vi "PWM_Mearsurement.vi"() -> ()   [LabVIEW 2019]
uses:
  <vilib>/rvi/Emulation/niFpgaGetClockAttributes.vi
  <vilib>/rvi/Emulation/niFpgaSctlEmulationGetInTimedLoop.vi
  <vilib>/rvi/Emulation/niFpgaEmulationReportErrorSimple.vi
  <vilib>/rvi/eio/common/nirviEmuTemplateMethod_errors.vi
  <vilib>/rvi/Emulation/niFpgaCriticalErrorInLSC.vi
  <vilib>/eio/EIONode/EIONode.xnode
panel:
  out "波形图表 3":cluster{u32, u32}(graph)
  out "时钟信号个数 3":u32
  out "被测信号个数 3":u32
  in  "Count(Ticks) 3":u32=16 caption="计数器(滴答)"
  out "波形图表 2":cluster{u32, u32}(graph)
  out "被测信号个数 2":u32
  out "时钟信号个数 2":u32
  in  "Count(Ticks) 2":u32=16 caption="计数器(滴答)"
  out "被测信号个数":u32
  out "时钟信号个数":u32
  out "x+1":u32
  out "数值":u32
  in  "Count(Ticks)":u32=16 caption="计数器(滴答)"
  out "x-1":u32
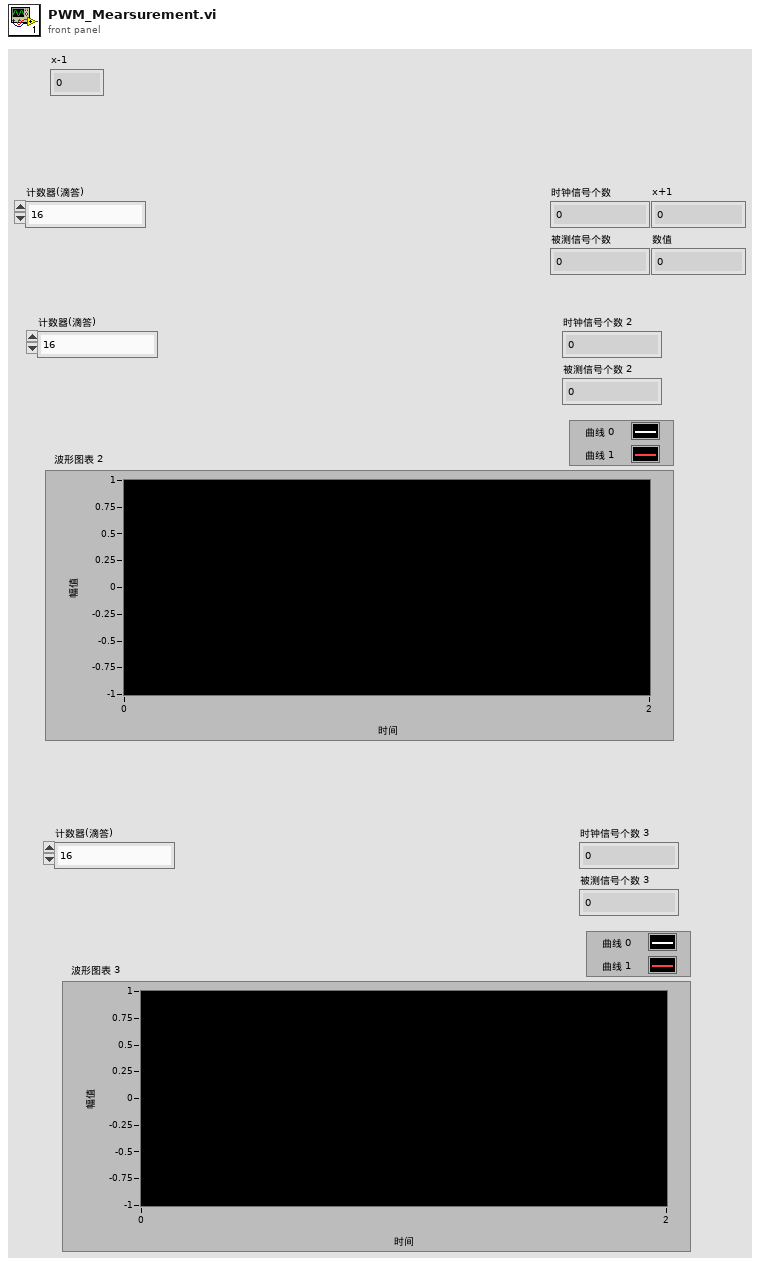
[diagram p1: front panel]
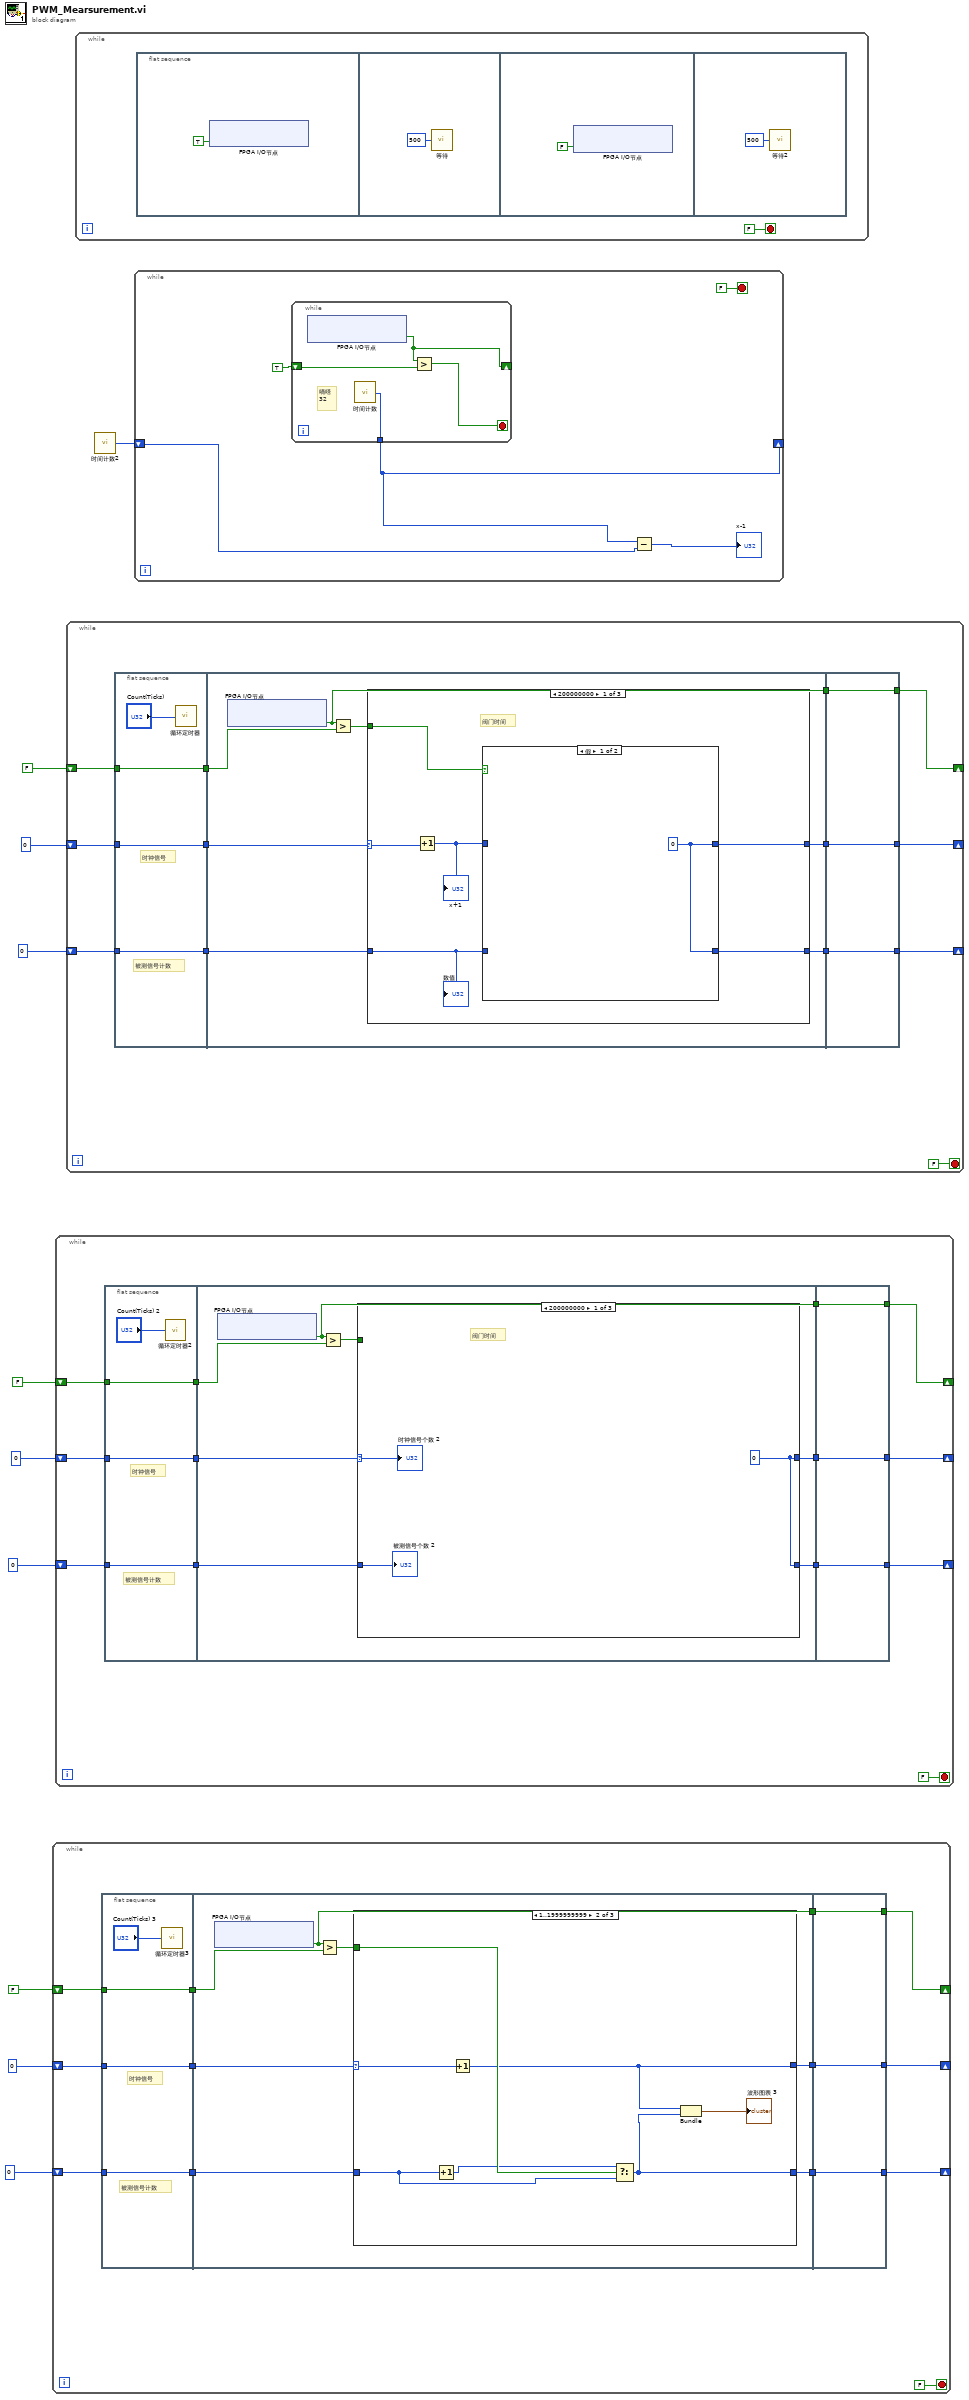
[diagram p0: block diagram]
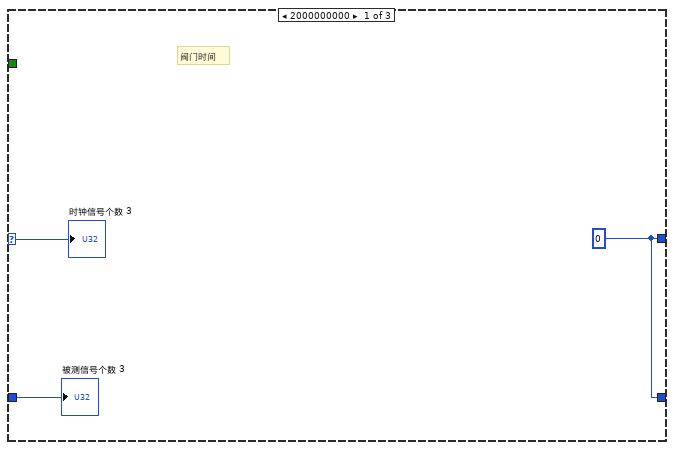
[diagram p2: hidden frame]
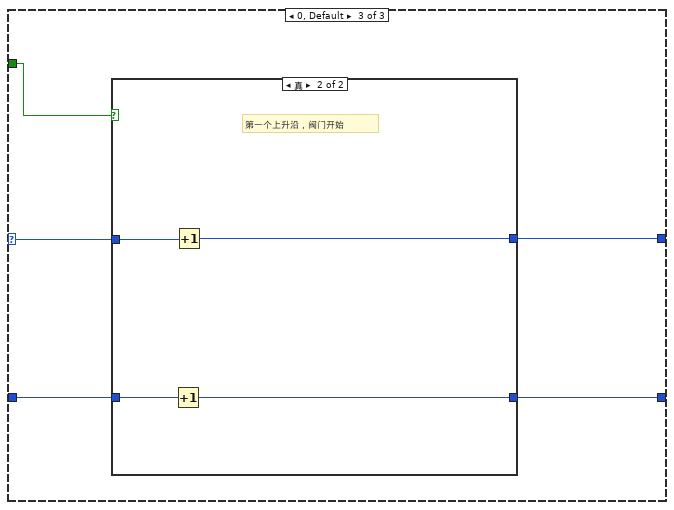
[diagram p3: hidden frame]
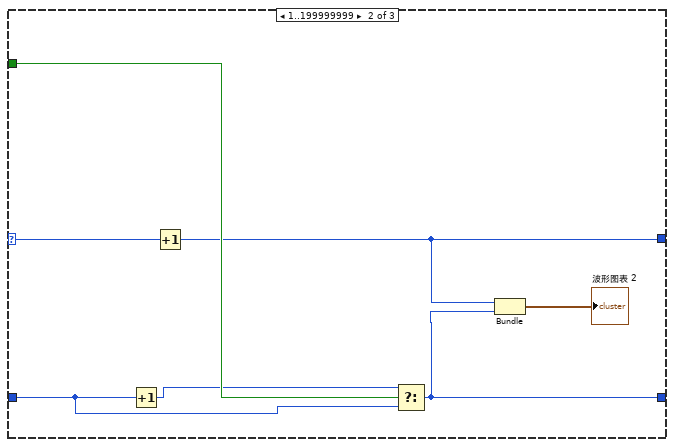
[diagram p5: hidden frame]
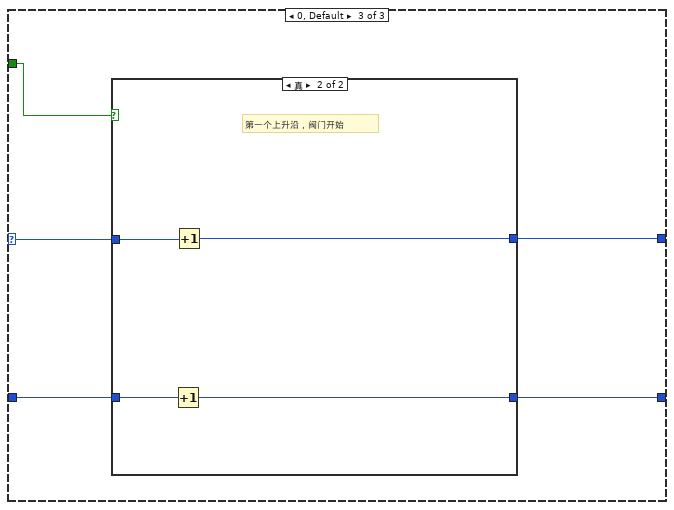
[diagram p6: hidden frame]
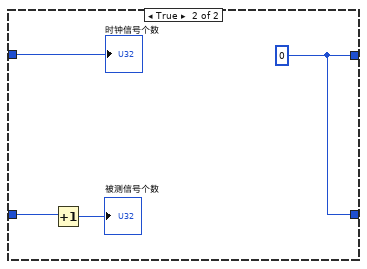
[diagram p8: hidden frame]
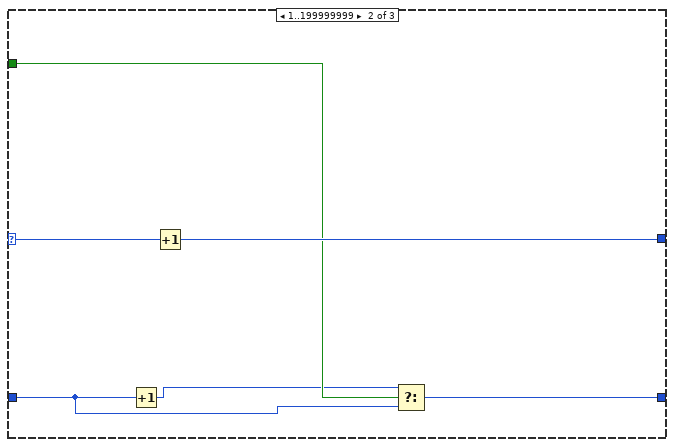
[diagram p9: hidden frame]
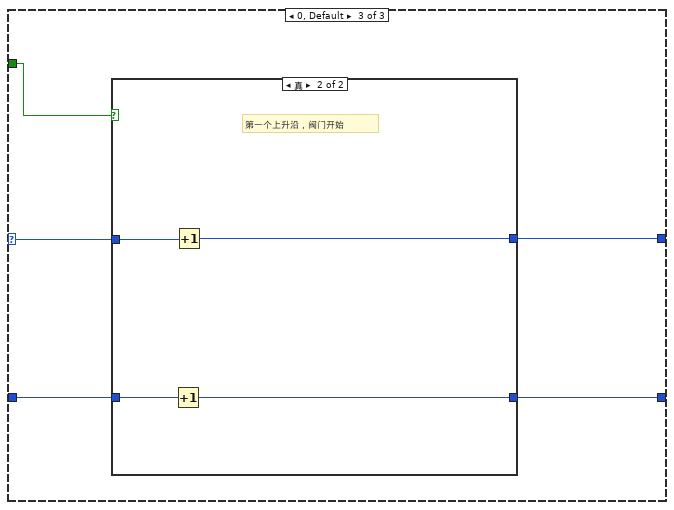
[diagram p10: hidden frame]
diagram:
  n1 = while {
    shift-right: [w14] -> _
    shift-left: FALSE -> [w21]
    shift-right: [w16] -> _
    shift-left: u32 0 -> [w19]
    shift-right: [w15] -> _
    shift-left: u32 0 -> [w17]
    stop <- FALSE stop-if-true
    n2 = flat-sequence {
      tunnel: [w26] -> w22
      tunnel: w21 -> [w26]
      tunnel: [w25] -> w20
      tunnel: w19 -> [w25]
      tunnel: [w24] -> w18
      tunnel: w17 -> [w24]
      tunnel: w22 -> [w34]
      tunnel: w20 -> [w33]
      tunnel: w18 -> [w31]
      tunnel: [w30] -> w13
      tunnel: [w29] -> w12
      tunnel: [w28] -> w11
      tunnel: [w56] -> w14
      tunnel: [w57] -> w15
      tunnel: [w58] -> w16
      tunnel: w13 -> [w58]
      tunnel: w12 -> [w57]
      tunnel: w11 -> [w56]
      frame #0 {
        # "被测信号计数"
        # "时钟信号"
        n3 = call "循环定时器3"("Count(Ticks)"="Count(Ticks) 3") -> ()  [unwired: 1 out]
      }
      frame #1 {
        n4 = xnode "FPGA I/O节点"() -> ("ConnectorB/DIO8"=w28:bool)  [unwired: 1 in, 1 out]
        n5 = Greater?(x=w28, y=w34) -> (0:w32:bool)
        n6 = case "条件结构" shown="1..1999999999" w33 {
          selector: w33 -> [w35 w44 w48]
          tunnel: w32 -> [_ w42 w49]
          tunnel: w31 -> [w36 w43 w47]
          tunnel: [w37 w41 w46] -> w30
          tunnel: [w37 w39 w45] -> w29
          frame 2000000000 {
            w37 = u32 0
            # "阀门时间"
            "时钟信号个数 3" <- w35
            "被测信号个数 3" <- w36
          }
          frame 1..1999999999 {
            n7 = Increment(x=w43) -> (x+1=w40:u32)
            n8 = Increment(x=w44) -> (x+1=w41:u32)
            n9 = Select(t=w40, s=w42, f=w43) -> (s? t:f=w39:u32)
            n10 = Bundle(w41, w39) -> (→"波形图表 3":cluster{u32, u32})  [unwired: 1 in]
          }
          frame 0, Default {
            n11 = case shown="真" w49 {
              tunnel: w48 -> [w51 w55]
              tunnel: w47 -> [w50 w54]
              tunnel: [w51 w53] -> w46
              tunnel: [w50 w52] -> w45
              frame False {
                # "不开始"
              }
              frame True {
                # "第一个上升沿，阀门开始"
                n12 = Increment(x=w54) -> (x+1=w52:u32)
                n13 = Increment(x=w55) -> (x+1=w53:u32)
              }
            }
          }
        }
      }
      frame #2 {
      }
    }
  }
  n14 = while {
    shift-right: [w62] -> _
    shift-left: FALSE -> [w69]
    shift-right: [w64] -> _
    shift-left: u32 0 -> [w67]
    shift-right: [w63] -> _
    shift-left: u32 0 -> [w65]
    stop <- FALSE stop-if-true
    n15 = flat-sequence {
      tunnel: [w74] -> w70
      tunnel: w69 -> [w74]
      tunnel: [w73] -> w68
      tunnel: w67 -> [w73]
      tunnel: [w72] -> w66
      tunnel: w65 -> [w72]
      tunnel: w70 -> [w82]
      tunnel: w68 -> [w81]
      tunnel: w66 -> [w79]
      tunnel: [w78] -> w61
      tunnel: [w77] -> w60
      tunnel: [w76] -> w59
      tunnel: [w104] -> w62
      tunnel: [w105] -> w63
      tunnel: [w106] -> w64
      tunnel: w61 -> [w106]
      tunnel: w60 -> [w105]
      tunnel: w59 -> [w104]
      frame #0 {
        # "被测信号计数"
        # "时钟信号"
        n16 = call "循环定时器2"("Count(Ticks)"="Count(Ticks) 2") -> ()  [unwired: 1 out]
      }
      frame #1 {
        n17 = xnode "FPGA I/O节点"() -> ("ConnectorB/DIO6"=w76:bool)  [unwired: 1 in, 1 out]
        n18 = Greater?(x=w76, y=w82) -> (0:w80:bool)
        n19 = case "条件结构" shown="200000000" w81 {
          selector: w81 -> [w83 w92 w96]
          tunnel: w80 -> [_ w90 w97]
          tunnel: w79 -> [w84 w91 w95]
          tunnel: [w85 w89 w94] -> w78
          tunnel: [w85 w87 w93] -> w77
          frame 200000000 {
            w85 = u32 0
            # "阀门时间"
            "时钟信号个数 2" <- w83
            "被测信号个数 2" <- w84
          }
          frame 1..199999999 {
            n20 = Increment(x=w91) -> (x+1=w88:u32)
            n21 = Increment(x=w92) -> (x+1=w89:u32)
            n22 = Select(t=w88, s=w90, f=w91) -> (s? t:f=w87:u32)
            n23 = Bundle(w89, w87) -> (→"波形图表 2":cluster{u32, u32})  [unwired: 1 in]
          }
          frame 0, Default {
            n24 = case shown="真" w97 {
              tunnel: w96 -> [w99 w103]
              tunnel: w95 -> [w98 w102]
              tunnel: [w99 w101] -> w94
              tunnel: [w98 w100] -> w93
              frame False {
                # "不开始"
              }
              frame True {
                # "第一个上升沿，阀门开始"
                n25 = Increment(x=w102) -> (x+1=w100:u32)
                n26 = Increment(x=w103) -> (x+1=w101:u32)
              }
            }
          }
        }
      }
      frame #2 {
      }
    }
  }
  n27 = while {
    shift-right: [w110] -> _
    shift-left: FALSE -> [w117]
    shift-right: [w112] -> _
    shift-left: u32 0 -> [w115]
    shift-right: [w111] -> _
    shift-left: u32 0 -> [w113]
    stop <- FALSE stop-if-true
    n28 = flat-sequence {
      tunnel: [w122] -> w118
      tunnel: w117 -> [w122]
      tunnel: [w121] -> w116
      tunnel: w115 -> [w121]
      tunnel: [w120] -> w114
      tunnel: w113 -> [w120]
      tunnel: w118 -> [w130]
      tunnel: w116 -> [w129]
      tunnel: w114 -> [w127]
      tunnel: [w126] -> w109
      tunnel: [w125] -> w108
      tunnel: [w124] -> w107
      tunnel: [w159] -> w110
      tunnel: [w160] -> w111
      tunnel: [w161] -> w112
      tunnel: w109 -> [w161]
      tunnel: w108 -> [w160]
      tunnel: w107 -> [w159]
      frame #0 {
        # "被测信号计数"
        # "时钟信号"
        n29 = call "循环定时器"("Count(Ticks)"="Count(Ticks)") -> ()  [unwired: 1 out]
      }
      frame #1 {
        n30 = xnode "FPGA I/O节点"() -> ("ConnectorB/DIO4"=w124:bool)  [unwired: 1 in, 1 out]
        n31 = Greater?(x=w124, y=w130) -> (0:w128:bool)
        n32 = case "条件结构" shown="200000000" w129 {
          selector: w129 -> [w135 w147 w151]
          tunnel: w128 -> [w136 w145 w152]
          tunnel: w127 -> [w134 w143 w150]
          tunnel: [w133 w146 w149] -> w126
          tunnel: [w132 w142 w148] -> w125
          frame 200000000 {
            # "阀门时间"
            n33 = Increment(x=w135) -> (x+1=w131:u32)
            "x+1" <- w131
            n34 = case shown="假" w136 {
              tunnel: w134 -> [_ w140]
              tunnel: [w137 w141] -> w133
              tunnel: [w137 w141] -> w132
              tunnel: w131 -> [_ w138]
              frame False {
                w137 = u32 0
              }
              frame True {
                w141 = u32 0
                n35 = Increment(x=w140) -> (x+1=→"被测信号个数":u32)
                "时钟信号个数" <- w138
              }
            }
            "数值" <- w134
          }
          frame 1..199999999 {
            n36 = Increment(x=w143) -> (x+1=w144:u32)
            n37 = Increment(x=w147) -> (x+1=w146:u32)
            n38 = Select(t=w144, s=w145, f=w143) -> (s? t:f=w142:u32)
          }
          frame 0, Default {
            n39 = case shown="真" w152 {
              tunnel: w151 -> [w154 w158]
              tunnel: w150 -> [w153 w157]
              tunnel: [w154 w156] -> w149
              tunnel: [w153 w155] -> w148
              frame False {
                # "不开始"
              }
              frame True {
                # "第一个上升沿，阀门开始"
                n40 = Increment(x=w157) -> (x+1=w155:u32)
                n41 = Increment(x=w158) -> (x+1=w156:u32)
              }
            }
          }
        }
      }
      frame #2 {
      }
    }
  }
  n42 = while {
    stop <- FALSE stop-if-true
    n43 = flat-sequence {
      frame #0 {
        n44 = xnode "FPGA I/O节点"("ConnectorB/DIO0"=TRUE ("ConnectorA/DIO0")) -> ()  [unwired: 1 in, 1 out]
      }
      frame #1 {
        n45 = call "等待"("Count(uSec)"=u32 500) -> ()  [unwired: 1 out]
      }
      frame #2 {
        n46 = xnode "FPGA I/O节点"("ConnectorB/DIO0"=FALSE ("ConnectorA/DIO0")) -> ()  [unwired: 1 in, 1 out]
      }
      frame #3 {
        n47 = call "等待2"("Count(uSec)"=u32 500) -> ()  [unwired: 1 out]
      }
    }
  }
  n48 = call "时间计数2"() -> ("Tick Count(Ticks)"=w10:u32)
  n49 = while {
    shift-right: [w169] -> _
    shift-left: w10 -> [w168]
    stop <- FALSE stop-if-true
    n50 = while {
      shift-right: [w174] -> _
      shift-left: TRUE -> [w175]
      tunnel: [w172] -> w169
      stop <- w173 stop-if-true
      # "嘀嗒\n32"
      n51 = xnode "FPGA I/O节点"() -> ("ConnectorB/DIO2"=w174:bool)  [unwired: 1 in, 1 out]
      n52 = call "时间计数"() -> ("Tick Count(Ticks)"=w172:u32)
      n53 = Greater?(x=w174, y=w175) -> (0:w173:bool)
    }
    n54 = Subtract(x=w169, y=w168) -> (x-y=→"x-1":u32)
  }
